vi "exampleClient.vi"() -> ()   [LabVIEW 2017]
uses:
  <vilib>/httpClient/POSTBuffer.vi
  <vilib>/httpClient/LabVIEWHTTPClient.lvlib
panel:
  out "response":string
  in  "Send":bool
  in  "Stop Button":bool
  in  "cmd":string
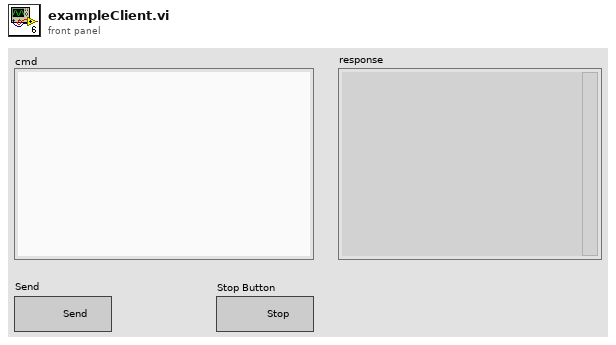
[diagram p1: front panel]
types:
  T1 = typedef "LabVIEWHTTPClient.lvlib/ClientHandle.ctl" = refnum<k1>
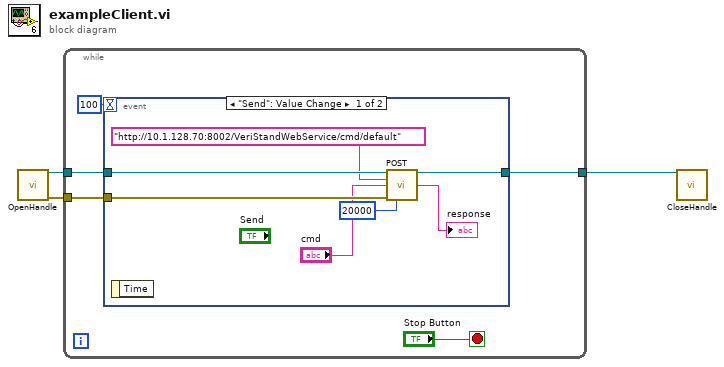
[diagram p0: block diagram]
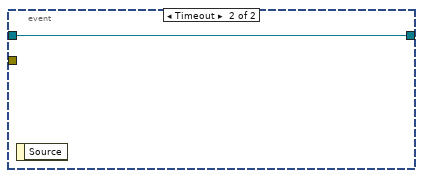
[diagram p2: hidden frame]
diagram:
  n1 = call <vilib>:"OpenHandle.vi"() -> ("client handle out"=w3:T1, "error out"=w2:errorcluster)  [unwired: 14 in]
  n2 = while {
    tunnel: w3 -> [w8]
    tunnel: w2 -> [w7]
    tunnel: [w6] -> w1
    stop <- "Stop Button" stop-if-true
    n3 = event shown="[0] \"Send\": Value Change" {
      selector: _ -> [_ _]
      dyn-events: _ -> [_ _]
      timeout: 100 -> [_ _]
      tunnel: w8 -> [w15 w16]
      tunnel: w7 -> [w14 _]
      tunnel: [w11 w16] -> w6
      event "Send": Value Change {
        n4 = event-data() -> ()  [unwired: 1 in, 1 out]
        n5 = call-poly <vilib>:"POST.vi"("client handle"=w15, "url"="http://10.1.128.70:8002/VeriStandWebService/cmd/default", "buffer"="cmd", "error in (no error)"=w14, "timeout (10000)"=20000) -> ("client handle out"=w11:T1, "body"=→"response":string)  [unwired: 7 in, 2 out]
      }
      event Timeout {
        n6 = event-data() -> ()  [unwired: 1 in, 1 out]
      }
    }
  }
  n7 = call <vilib>:"CloseHandle.vi"("client handle"=w1) -> ()  [unwired: 14 in, 1 out]
